vi "mxwScript_API_XMLConvertToLocal.vi"(8 "error in (no error)":errorcluster, 10 "read/write":T1="Auto", 11 "controlToLinkTo":string) -> (0 "error out":errorcluster, 3 "encoded connectorPaneName":string)   [LabVIEW 2017]
doc: "Create encoded \"connectorPaneName\" for converting a control to a local variable."
uses:
  codeGenAPISupport.llb/cgAPI_mxwScript_ConnPaneConvertToLocalType.ctl
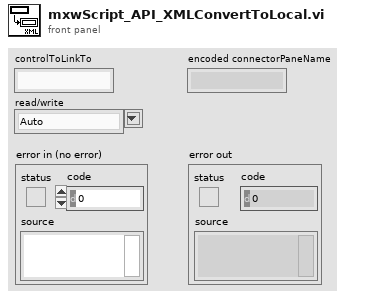
[diagram p1: front panel]
types:
  T1 = typedef "cgAPI_mxwScript_ConnPaneConvertToLocalType.ctl" = string
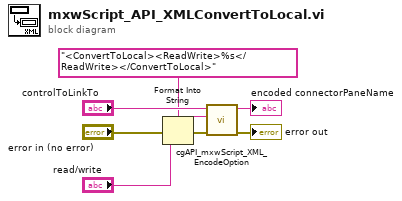
[diagram p0: block diagram]
diagram:
  n1 = Format Into String(format string="<ConvertToLocal><ReadWrite>%s</ReadWrite></ConvertToLocal>" ("control name"), error in="error in (no error)", "read/write") -> (resulting string=w3:string, error out=w5:errorcluster)  [unwired: 1 in]
  n2 = call "cgAPI_mxwScript_XML_EncodeOption.vi"("error in (no error)"=w5, "otherXML"=w3, "normalTextString"="controlToLinkTo") -> ("error out"=→"error out":errorcluster, "encodedString"=→"encoded connectorPaneName":string)  [unwired: 7 out]
